vi "SerialTest.vi"() -> ()   [LabVIEW 2009]
uses:
  Serial.lvlib
panel:
  out "data out":u8[](array[numeric])
  out "Message ID Out":u32 format="%x"
  in  "data":u8[](array[numeric])
  in  "messageID":u32 format="%.0x"
  out "error out":errorcluster
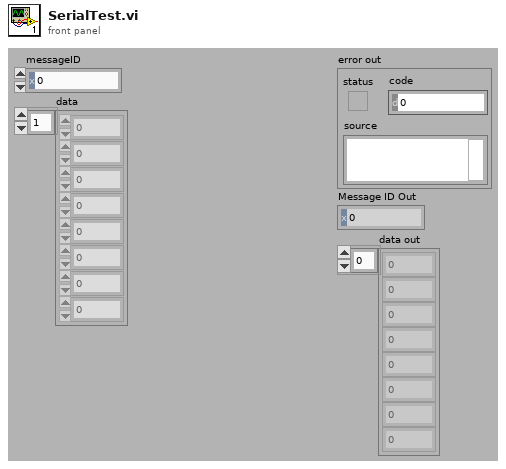
[diagram p1: front panel]
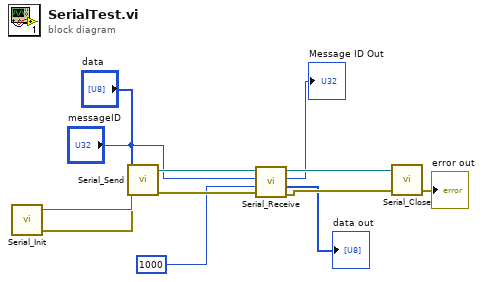
[diagram p0: block diagram]
diagram:
  n1 = call "Serial_Init.vi"() -> ("error out"=w11:errorcluster, "VISA resource name out"=w12:refnum<visa-resource-name>)  [unwired: 4 in]
  n2 = call "Serial_Send.vi"("error in"=w11, "data"="data", "messageID"="messageID", "VISA resource name"=w12) -> ("error out"=w9:errorcluster, "VISA resource name out"=w6:refnum<visa-resource-name>)  [unwired: 6 in]
  n3 = call "Serial_Receive.vi"("error in (no error)"=w9, "timeoutMs"=u32 1000, "Message ID"="messageID", "VISA resource name"=w6) -> ("error out"=w8:errorcluster, "data"=→"data out":u8[], "Message ID Out"=→"Message ID Out":u32, "VISA resource name out"=w7:refnum<visa-resource-name>)  [unwired: 4 in]
  n4 = call "Serial_Close.vi"("error in (no error)"=w8, "VISA resource name"=w7) -> ("error out"=→"error out":errorcluster)  [unwired: 3 in]
